vi "ShootTest.vi"(0 "Shoot during x ms":dbl, 1 "Arduino Serial Port":refnum<visa-resource-name>, 2 "error in (no error)":errorcluster caption="entrée d'erreur (pas d'erreur)") -> (3 "Arduino Serial out":refnum<visa-resource-name>, 4 "Message":string, 5 "Shot Until":dbl, 6 "error out":errorcluster caption="sortie d'erreur")   [LabVIEW 2014, in "ShootingStar.lvlib"]
uses:
  <vilib>/Instr/_visa.llb/VISA Configure Serial Port (Instr).vi
  ShootingStar.lvlib
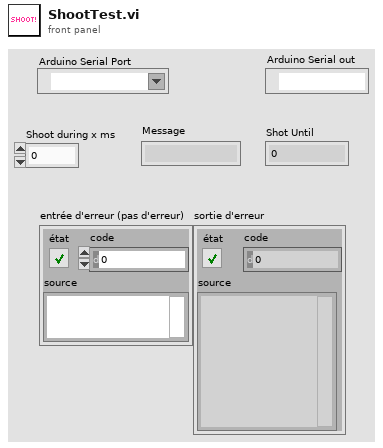
[diagram p1: front panel]
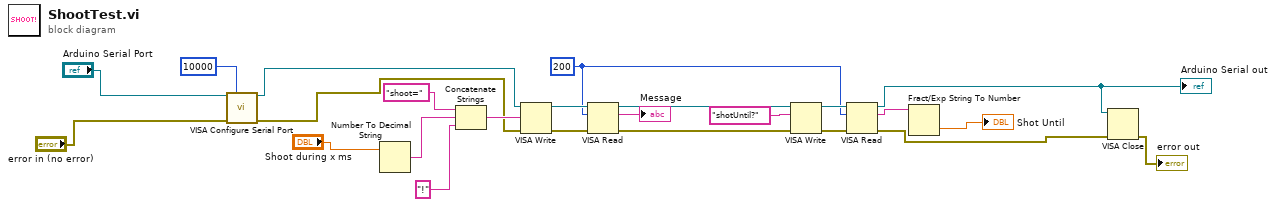
[diagram p0: block diagram]
diagram:
  w17 = u32 200 ("nombre d'octets")
  n1 = call-poly "VISA Configure Serial Port"("VISA resource name"="Arduino Serial Port", "timeout (10sec)"=u32 10000, "error in (no error)"="error in (no error)") -> ("VISA resource name out"=w2:refnum<visa-resource-name>, "error out"=w1:errorcluster)  [unwired: 11 in]
  n2 = Number To Decimal String(number="Shoot during x ms") -> (decimal integer string=w11:string)  [unwired: 1 in]
  n3 = Concatenate Strings("shoot=" ("buffer à écrire"), w11, "!") -> (w10:string)
  n4 = VISA Write(VISA resource name=w2, write buffer=w10, error in (no error)=w1) -> (VISA resource name out=w24:refnum<visa-resource-name>, error out=w23:errorcluster)  [unwired: 1 out]
  n5 = VISA Read(VISA resource name=w24, byte count=w17, error in (no error)=w23) -> (VISA resource name out=w21:refnum<visa-resource-name>, read buffer=→"Message":string, error out=w20:errorcluster)  [unwired: 1 out]
  n6 = VISA Write(VISA resource name=w21, write buffer="shotUntil?", error in (no error)=w20) -> (VISA resource name out=w18:refnum<visa-resource-name>, error out=w16:errorcluster)  [unwired: 1 out]
  n7 = VISA Read(VISA resource name=w18, byte count=w17, error in (no error)=w16) -> (VISA resource name out=w3:refnum<visa-resource-name>, read buffer=w15:string, error out=w5:errorcluster)  [unwired: 1 out]
  "Arduino Serial out" <- w3
  n8 = Fract/Exp String To Number(string=w15) -> (number=→"Shot Until":dbl)  [unwired: 3 in, 1 out]
  n9 = VISA Close(VISA resource name=w3, error in (no error)=w5) -> (error out=→"error out":errorcluster)
